vi "Update Sort Column.vi"(6 "Reset?":bool, 8 "error in":errorcluster, 10 "Cell Position":T1, 11 "Peer Review in":refnum<class "Peer Review.lvclass">) -> (0 "error out":errorcluster, 3 "Peer Review out":refnum<class "Peer Review.lvclass">)   [LabVIEW 2020, in "Peer Review.lvclass"]
uses:
  Peer Review.lvclass
  <vilib>/Utility/miscctls.llb/LVRowAndColumnTypeDef.ctl
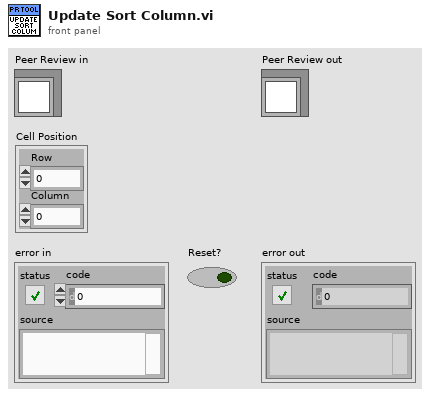
[diagram p1: front panel]
types:
  T1 = typedef "LVRowAndColumnTypeDef.ctl" = cluster{"Row":i32, "Column":i32}
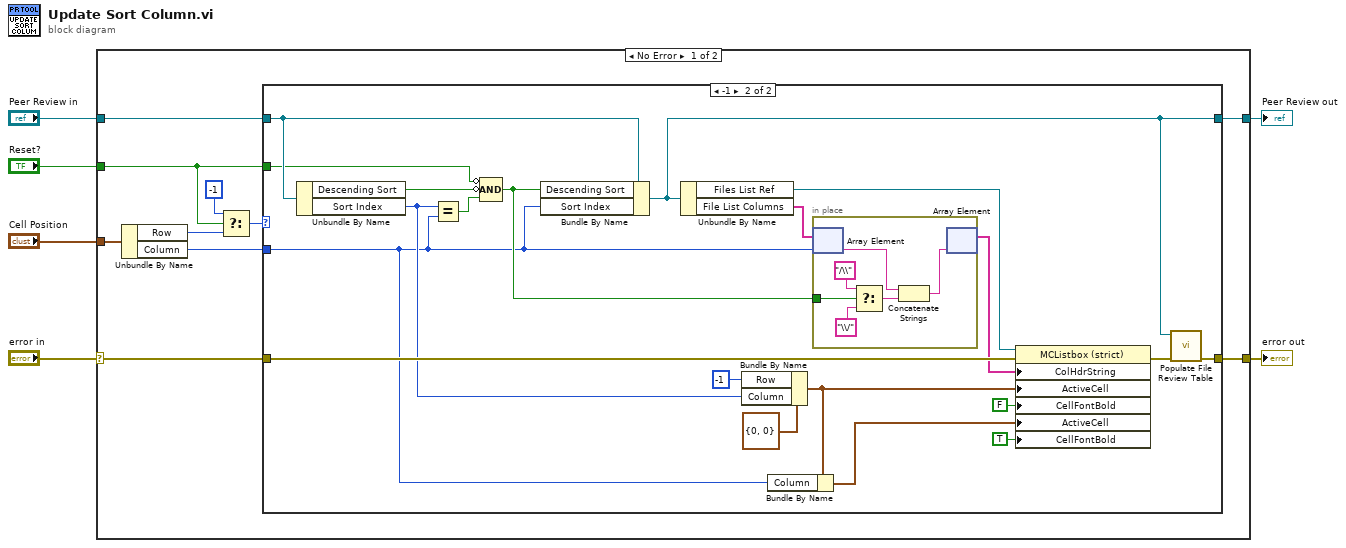
[diagram p0: block diagram]
diagram:
  n1 = case shown="No Error" "error in" {
    selector: "error in" -> [w11 w46]
    tunnel: [w16 w46] -> w5
    tunnel: "Cell Position" -> [w12 _]
    tunnel: "Peer Review in" -> [w14 w45]
    tunnel: [w13 w45] -> w2
    tunnel: "Reset?" -> [w10 _]
    frame No Error {
      n2 = Unbundle By Name(w12) -> ("Row"=w8:i32, "Column"=w15:i32)
      n3 = Select(t=-1, s=w10, f=w8) -> (s? t:f=w7:i32)
      n4 = case shown="-1" w7 {
        tunnel: [w18 w23] -> w16
        tunnel: w11 -> [w18 w34]
        tunnel: w15 -> [_ w20]
        tunnel: w14 -> [w17 w28]
        tunnel: [w17 w19] -> w13
        tunnel: w10 -> [_ w22]
        frame Default {
          # "Not a column header, so do nothing."
        }
        frame -1 {
          n5 = Unbundle By Name(w28) -> ("Descending Sort"=w29:bool, "Sort Index"=w30:i32)
          n6 = Equal?(x=w30, y=w20) -> (x = y?=w32:bool)
          n7 = Compound Arithmetic op=AND(invert w22, invert w29, w32) -> (w21:bool)
          n8 = Bundle By Name(cluster=w28, "Descending Sort"=w21, "Sort Index"=w20) -> (w19:refnum<class "Peer Review.lvclass">)
          n9 = Unbundle By Name(w19) -> ("Files List Ref"=w27:refnum<vi>, "File List Columns"=w26:string[])
          n10 = Bundle By Name(cluster=T1 {"Row"=0, "Column"=0} ("Active Cell:Active Cell"), "Row"=-1, "Column"=w30) -> (w33:T1)
          n11 = Bundle By Name(cluster=w33, "Column"=w20) -> (w25:T1)
          n12 = in-place {
            in-place-border: w21 -> [w41]
            n13 = in-place-array #1(w26, w20) -> (w40:string)
            n14 = Select(t="/\\" ("y"), s=w41, f="\\/" ("y")) -> (s? t:f=w44:string)
            n15 = Concatenate Strings(w40, w44) -> (w39:string)
            n16 = in-place-array #1(w39) -> (w31:string[])  [unwired: 1 out]
          }
          n17 = property on="Property Node" class="MCListbox (strict)"(reference=w27, error in=w34, "ColHdrString"=w31, "ActiveCell"=w33, "CellFontBold"=FALSE ("Active Cell:Cell Font:Bold"), "ActiveCell"=w25, "CellFontBold"=TRUE ("Active Cell:Cell Font:Bold")) -> (error out=w24:errorcluster)  [unwired: 1 out]
          n18 = call "Populate File Review Table.vi"("error in"=w24, "Peer Review"=w19) -> ("error out"=w23:errorcluster)  [unwired: 9 in]
        }
      }
    }
    frame Error {
    }
  }
  "error out" <- w5
  "Peer Review out" <- w2
